vi "Create_QR_folder.vi"(9 "name or relative path":string, 11 "扭力曲線位置":path) -> (2 "Curve存放位置":path)   [LabVIEW 2019]
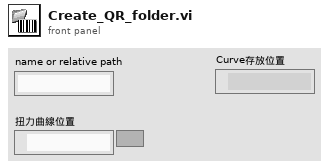
[diagram p1: front panel]
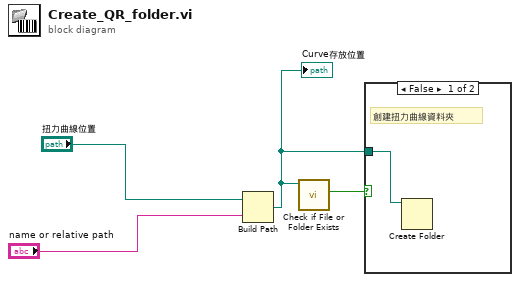
[diagram p0: block diagram]
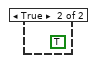
[diagram p2: hidden frame]
diagram:
  n1 = Build Path(base path="扭力曲線位置", name or relative path="name or relative path") -> (appended path=w3:path)
  "Curve存放位置" <- w3
  n2 = call <vilib>:"Check if File or Folder Exists.vi"("path"=w3) -> ("file or folder exists?"=w2:bool)  [unwired: 8 in, 2 out]
  n3 = case shown="False" w2 {
    tunnel: w3 -> [w5 _]
    frame False {
      # "創建扭力曲線資料夾"
      n4 = Create Folder(path (use dialog)=w5) -> ()  [unwired: 2 in, 3 out]
    }
    frame True {
      (unwired) TRUE ("主資料夾")
    }
  }
